vi "IPS120_stamp.vi"(1 "in":string) -> (0 "out":string)   [LabVIEW 2012]
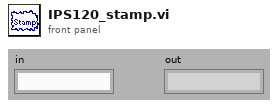
[diagram p1: front panel]
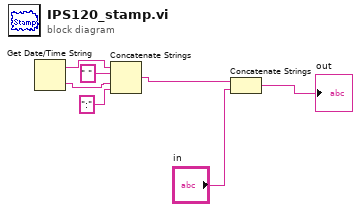
[diagram p0: block diagram]
diagram:
  n1 = Get Date/Time String() -> (date string=w1:string, time string=w3:string)  [unwired: 3 in]
  n2 = Concatenate Strings(w1, " " ("string"), w3, ":" ("string")) -> (w5:string)
  n3 = Concatenate Strings(w5, "in") -> (→"out":string)
